vi "Finalize.vi"(8 "error in (no error)":errorcluster, 11 "Zenoh in":refnum<class "Zenoh.lvclass">) -> (0 "error out":errorcluster, 3 "Zenoh out":refnum<class "Zenoh.lvclass">)   [LabVIEW 2021, in "Zenoh.lvclass"]
uses:
  Zenoh.lvclass
  Zenoh.lvclass/Zenoh.ctl
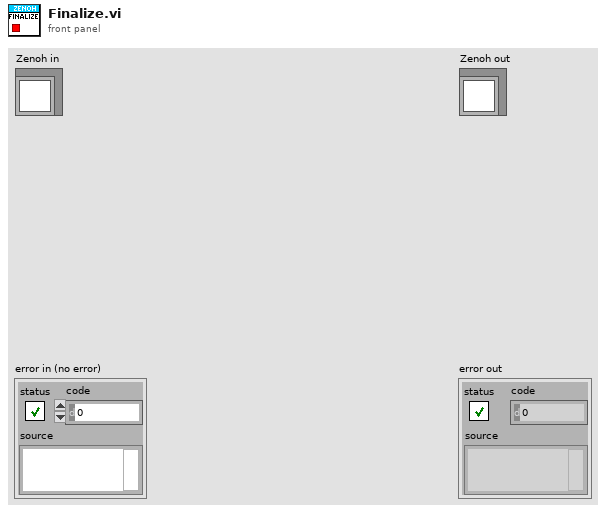
[diagram p1: front panel]
types:
  T1 = typedef "Zenoh.lvclass/Channel Info.ctl" = cluster{"Mime Type":string, "Reader Handle":u64}
  T2 = typedef "Zenoh.lvclass/Storage Info.ctl" = cluster{"Storage Handle":u64}
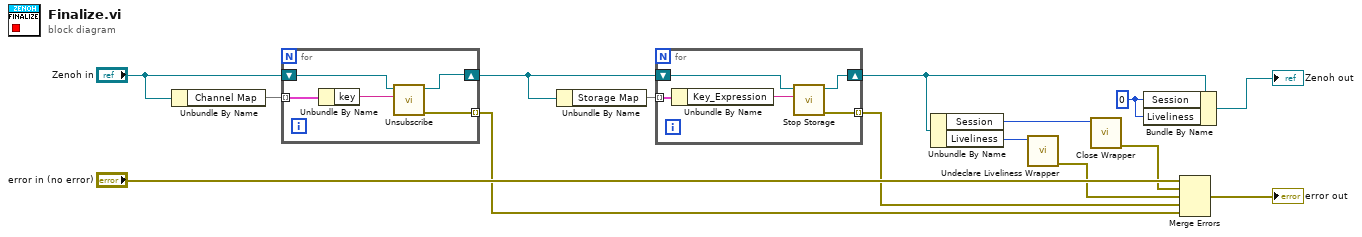
[diagram p0: block diagram]
diagram:
  w6 = u64 0 ("Session")
  n1 = Unbundle By Name("Zenoh in") -> ("Channel Map"=w15:map{string, T1})
  n2 = for {
    tunnel: w15 -> [w20] mode=indexing
    shift-right: [w17] -> w4
    shift-left: "Zenoh in" -> [w18]
    tunnel: [w16] -> w2 mode=indexing
    n3 = Unbundle By Name(w20) -> ("key"=w19:string)
    n4 = call "Unsubscribe.vi"("Key"=w19, "Zenoh in"=w18) -> ("error out"=w16:errorcluster, "Zenoh out"=w17:refnum<class "Zenoh.lvclass">)  [unwired: 8 in]
  }
  n5 = Unbundle By Name(w4) -> ("Storage Map"=w5:map{string, T2})
  n6 = for {
    tunnel: w5 -> [w25] mode=indexing
    shift-right: [w21] -> w3
    shift-left: w4 -> [w22]
    tunnel: [w23] -> w1 mode=indexing
    n7 = Unbundle By Name(w25) -> ("Key_Expression"=w24:string)
    n8 = call "Stop Storage.vi"("Key Expression"=w24, "Zenoh in"=w22) -> ("error out"=w23:errorcluster, "Zenoh out"=w21:refnum<class "Zenoh.lvclass">)  [unwired: 8 in]
  }
  n9 = Unbundle By Name(w3) -> ("Session"=w14:u64, "Liveliness"=w8:u64)
  n10 = call "Undeclare Liveliness Wrapper.vi"("Liveliness Token"=w8) -> ("error out"=w7:errorcluster)  [unwired: 10 in]
  n11 = call "Close Wrapper.vi"("Session"=w14) -> ("error out"=w10:errorcluster)  [unwired: 10 in]
  n12 = Bundle By Name(cluster=w3, "Session"=w6, "Liveliness"=w6) -> (→"Zenoh out":refnum<class "Zenoh.lvclass">)
  n13 = Merge Errors("error in (no error)", w10, w7, w1, w2) -> (→"error out":errorcluster)
